vi "Main.vi"(11 "Module Admin":refnum<class "Delacor_lib_QMH_Cloneable Module Admin.lvclass">) -> ()   [LabVIEW 2020, in "Hardware Interface.lvlib"]
doc: "This template is based off of the Queued Message Handler design pattern and the Queued Message Handler project template that ships with LabVIEW.\n\nThe main difference is that the queue is private to this module and communication between modules is performed via Broadcast and Request events.\n\nRequest events are wrapped in public API methods and are handled in the Event Handling Loop (EHL) of this VI. Any module can register for Broadcast events sent by this module. The EHL generates messages based on user interface actions.\n\nThe Message Handling Loop (MHL) processes messages generated by the EHL, or by other messages. The messages are string values, so new messages can be added easily to the Message Cases case structure in the MHL. Each message cluster can also provide an optional value for Message Data, which is a variant that can be converted to whatever message-specific data is required.\n_____\nBased on Delacor QMH Project Template 5.0.0.82."
uses:
  Hardware Interface.lvlib
  <vilib>/Delacor/Delacor QMH/Libraries/Cloneable Module Admin_class/Delacor_lib_QMH_Cloneable Module Admin.lvclass
  C:/Program Files (x86)/National Instruments/LabVIEW 2020/vi.lib/Delacor/Delacor QMH/Libraries/Module Admin_class/Delacor_lib_QMH_Module Admin.lvclass
  Module Data--cluster.ctl
  MCU/MCU.lvclass
  <vilib>/Delacor/Delacor QMH/Libraries/Cloneable Module Admin_class/Delacor_lib_QMH_Cloneable Module Admin.lvclass/Delacor_lib_QMH_Cloneable Module Admin.ctl
  Stop Argument--cluster.ctl
  <vilib>/Delacor/Delacor QMH/Libraries/Message Queue_class/Delacor_lib_QMH_Message Queue.lvclass/Delacor_lib_QMH_Message Queue.ctl
  <vilib>/Delacor/Delacor QMH/Libraries/Module Admin_class/Delacor_lib_QMH_Module Admin.lvclass/Delacor_lib_QMH_Module Admin.ctl
  Serial Device Init Argument--cluster.ctl
  SetPort Argument--cluster.ctl
  <vilib>/Delacor/Delacor QMH/Libraries/Cloneable Module Admin_class/Delacor_lib_QMH_Get Module ID.vi
  <vilib>/Delacor/Delacor QMH/Libraries/Message Queue_class/Delacor_lib_QMH_Enqueue Message (Single).vi
  <vilib>/Delacor/Delacor QMH/Libraries/Module Admin_class/Delacor_lib_QMH_Get External Launch.vi
  <vilib>/Utility/error.llb/Error Cluster From Error Code.vi
  <vilib>/ErrorRing/Error Ring.xnode
  <vilib>/Delacor/Delacor QMH/Libraries/Message Queue_class/Delacor_lib_QMH_Message Queue.lvclass
panel:
  in  "Canal de ADC":u8
  in  "Update ADC":bool
  out "ADC":u16(knob) caption="Gauge" scale=0.0..4095.0
  in  "Pin a leer":u8
  in  "Adquirir Pin":bool
  out "Estado de pin":bool
  in  "Puerto a leer":u8
  in  "Adquirir Puerto":bool
  out "Salida de Puerto":bool[](array[boolean])
  in  "Entrada de Pin":bool
  in  "Escribir Pin":bool
  in  "Pin":u8
  in  "Puerto":u8
  in  "Escribir Puerto":bool
  in  "Entrada de Puerto":bool[](array[boolean])
  out "error out":errorcluster
  out "Status":string
  # "Hardware Abstraction Layer Example"
  # "Developed by Francisco Flores"
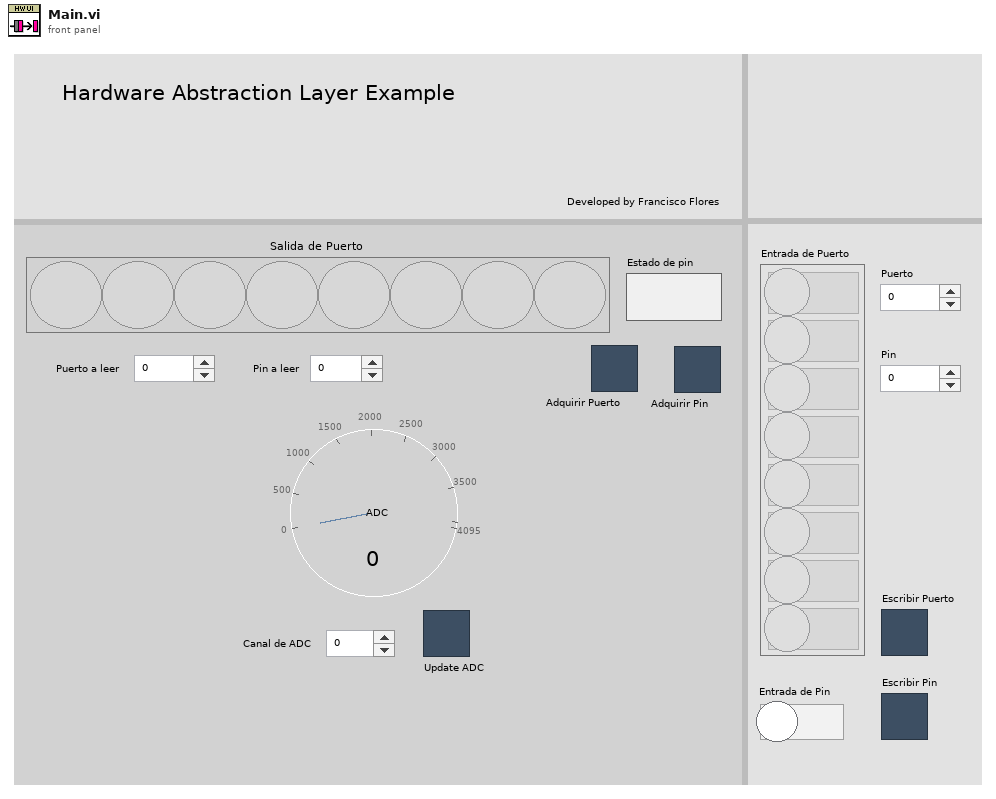
[diagram p1: front panel]
types:
  T1 = typedef "Hardware Interface.lvlib/Request Events--cluster.ctl" = cluster{"Stop Module":refnum<user-event>, "Show Panel":refnum<user-event>, "Hide Panel":refnum<user-event>, "Show Diagram":refnum<user-event>, "Get Module Execution Status":refnum<user-event>, "Serial Device Init":refnum<user-event>, "SetPort":refnum<user-event>}
  T2 = typedef "Hardware Interface.lvlib/Module Data--cluster.ctl" = cluster{"Status":string, "MCU.lvclass":refnum<class "MCU.lvclass">}
  T3 = enum32{"invalid lock state", "Not Locked", "Locked (No Password)", "Password-protected"}
  T4 = typedef "Hardware Interface.lvlib/Stop Argument--cluster.ctl" = cluster{"Module ID":i32, "Origin":string, "Exit via Stop Module Req?":bool, "Wait for Module to stop?":bool}
  T5 = typedef "Hardware Interface.lvlib/Serial Device Init Argument--cluster.ctl" = cluster{"Module ID":i32, "MCU.lvclass":refnum<class "MCU.lvclass">}
  T6 = typedef "Hardware Interface.lvlib/SetPort Argument--cluster.ctl" = cluster{"Module ID":i32, "Data":bool[], "Port":u8}
  T7 = enum32{"Invalid", "Standard", "Closed", "Hidden", "Minimized", "Maximized"}
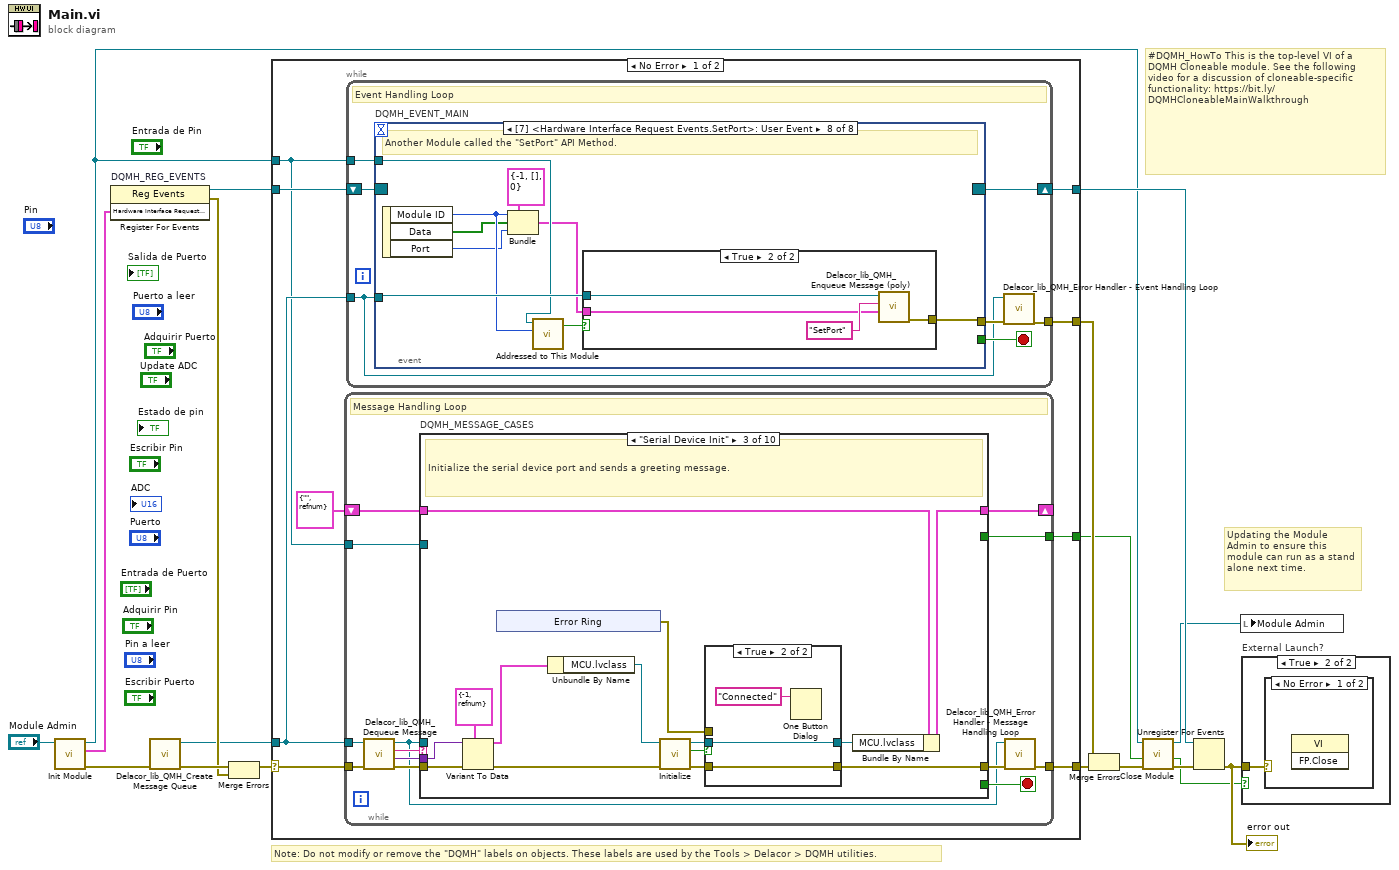
[diagram p0: block diagram]
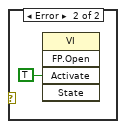
[diagram p3: hidden frame]
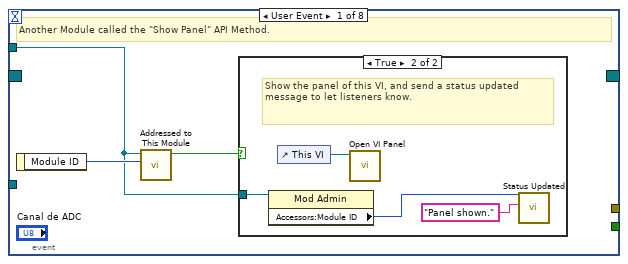
[diagram p4: hidden frame]
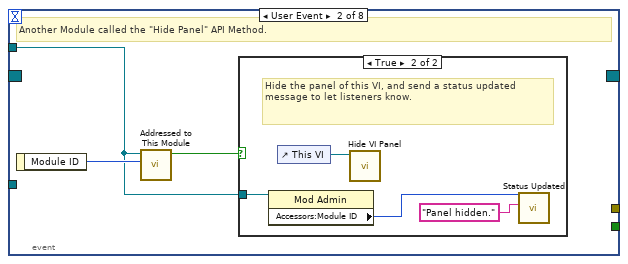
[diagram p6: hidden frame]
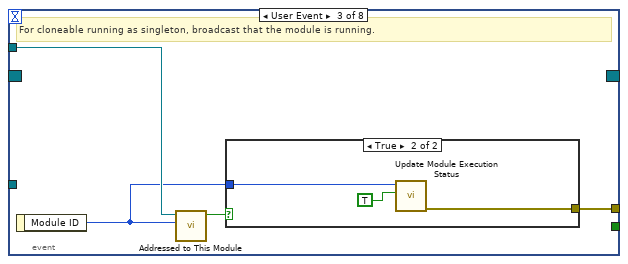
[diagram p8: hidden frame]
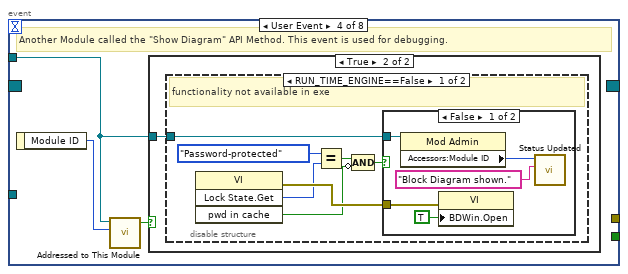
[diagram p10: hidden frame]
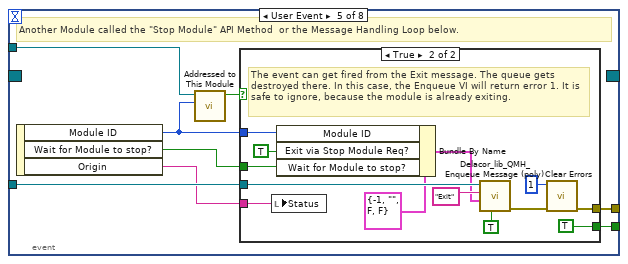
[diagram p14: hidden frame]
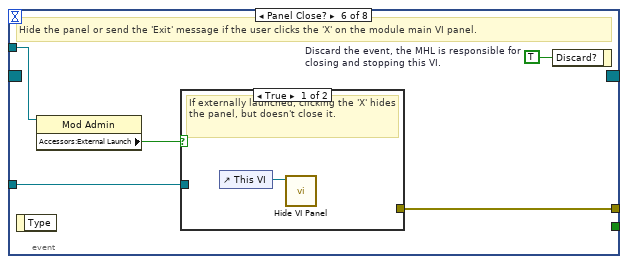
[diagram p16: hidden frame]
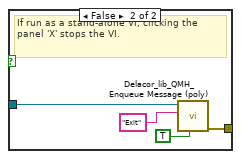
[diagram p17: hidden frame]
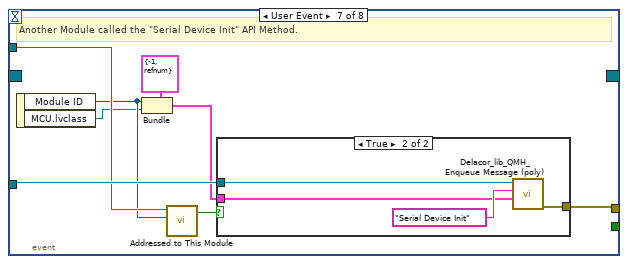
[diagram p18: hidden frame]
diagram:
  # "#DQMH_HowTo This is the top-level VI of a DQMH Cloneable module. See the following video for a discussion of cloneable-specific functionality: https://bit.ly/DQMHCloneableMainWalkthrough"
  # "Note: Do not modify or remove the \"DQMH\" labels on objects. These labels are used by the Tools > Delacor > DQMH utilities."
  # "Updating the Module Admin to ensure this module can run as a stand alone next time."
  n1 = call "Init Module.vi"("Cloneable Module Admin in"="Module Admin") -> ("error out"=w15:errorcluster, "Hardware Interface Request Events"=w7:T1, "Cloneable Module Admin out"=w4:refnum<class "Delacor_lib_QMH_Cloneable Module Admin.lvclass">)  [unwired: 8 in]
  n2 = register-events "DQMH_REG_EVENTS"(w7) -> (reference out=w8:refnum<event-registration>, error out=w10:errorcluster)  [unwired: 2 in]
  n3 = call <vilib>:"Delacor_lib_QMH_Create Message Queue.vi"("error in (no error)"=w15) -> ("error out"=w12:errorcluster, "Message Queue"=w6:refnum<class "Delacor_lib_QMH_Message Queue.lvclass">)  [unwired: 9 in]
  n4 = Merge Errors(w12, w10) -> (w11:errorcluster)
  n5 = case shown="No Error" w11 {
    selector: w11 -> [w25 w273]
    tunnel: [w27 w272] -> w16
    tunnel: [w24 w280] -> w9
    tunnel: w8 -> [w22 w280]
    tunnel: w6 -> [w21 w271]
    tunnel: [w26 _] -> w17
    tunnel: w4 -> [w20 w276]
    tunnel: [w19 _] -> w2
    frame No Error {
      n6 = while {
        tunnel: w21 -> [w131]
        shift-right: [w135] -> _
        shift-left: T2 {"Status"="", "MCU.lvclass"=refnum} ("Data Cluster") -> [w136]
        tunnel: w25 -> [w139]
        tunnel: [w137] -> w27
        tunnel: w20 -> [w129]
        tunnel: [w128] -> w19
        stop <- w134 stop-if-true
        # "Message Handling Loop"
        n7 = call-dynamic "Delacor_lib_QMH_Dequeue Message.vi"("error in (no error)"=w139, "Message Queue in"=w131) -> ("error out"=w138:errorcluster, "Message Data"=w132:variant, "Message"=w133:string, "Message Queue out"=w130:refnum<class "Delacor_lib_QMH_Message Queue.lvclass">)  [unwired: 6 in]
        n8 = case "DQMH_MESSAGE_CASES" shown="\"Serial Device Init\"" w133 {
          selector: w133 -> [_ _ _ _ _ _ _ _ _ w258]
          tunnel: w130 -> [_ _ _ _ _ _ w209 _ w248 _]
          tunnel: w138 -> [w158 w162 w176 w201 w204 w206 w218 w231 w254 w260]
          tunnel: [w156 w162 w166 w194 w203 w206 w214 w230 w251 w261] -> w140
          tunnel: w136 -> [w149 w161 w175 w197 w202 w205 w213 w228 w247 w259]
          tunnel: [w148 w161 w165 w196 w202 w205 w213 w228 w247 w259] -> w135
          tunnel: [_ _ _ _ _ _ _ _ w246 _] -> w134
          tunnel: w132 -> [_ _ w174 w200 _ _ w212 _ w244 _]
          tunnel: w129 -> [w143 _ _ _ _ _ w211 w226 w240 w256]
          tunnel: [_ _ _ _ _ _ _ _ w242 _] -> w128
          frame "Initialize" {
            w141 = "Initial Message" ("Initial Message")
            # "#CodeNeeded - Initialize the appearance of the front panel."
            # "#CodeNeeded - Initialize your state data here."
            # "Initialize - Any operation that needs to be done before the module can receive messages. Synchronize Caller Events.vi will inform Start Module.vi that the module has launched and is ready to receive messages. Module Did Init.vi will broadcast that the module initialized."
            n9 = call "Synchronize Caller Events.vi"("error in (no error)"=w158, "Module Admin"=w143) -> ("error out"=w157:errorcluster, "Module Admin out"=w142:refnum<class "Delacor_lib_QMH_Cloneable Module Admin.lvclass">)  [unwired: 8 in]
            n10 = property class="Mod Admin"(reference=w142) -> ("Accessors:Module ID"=w145:i32, "Accessors:External Launch"=w144:bool)  [unwired: 1 in, 2 out]
            n11 = call "Module Name--constant.vi"("Module ID"=w145) -> ("Module Name"=w153:string)  [unwired: 10 in]
            n12 = property class="VI"("Front Panel.Title"=w153) -> (reference out=w155:refnum<vi>, error out=w160:errorcluster)  [unwired: 2 in]
            n13 = Select(t=T7."Hidden" ("State"), s=w144, f=T7."Standard" ("State")) -> (s? t:f=w150:T7)
            n14 = invoke class="VI" method="FP.Open"(reference=w155, error in=w160, "State"=w150) -> (reference out=w154:refnum<vi>, error out=w159:errorcluster)  [unwired: 2 in, 3 out]
            n15 = call "Module Name--constant.vi"("Module ID"=w145) -> ("Module Name"=w146:string)  [unwired: 10 in]
            n16 = Bundle By Name(cluster=w149, "Status"=w141) -> (w148:T2)
            n17 = invoke class="VI" method="FP.Center"(reference=w154, error in=w159) -> ()  [unwired: 1 in, 3 out]
            n18 = call "Module Did Init.vi"("error in (no error)"=w157, "Initialized?"=TRUE, "Origin"=w146, "Module ID"=w145) -> ("error out"=w156:errorcluster)  [unwired: 7 in]
            "Status" <- w141
          }
          frame "--- Module Specific ---" {
            # "Separator -- The following cases handle messages specific to this Module."
          }
          frame "Serial Device Init" {
            # "Initialize the serial device port and sends a greeting message."
            n19 = Variant To Data(error in=w176, type=T5 {"Module ID"=-1, "MCU.lvclass"=refnum} ("Serial Device Init Argument"), Variant=w174) -> (data=w172:T5, error out=w171:errorcluster)
            n20 = xnode "Error Ring"() -> ("error out"=w163:errorcluster)
            n21 = Unbundle By Name(w172) -> ("MCU.lvclass"=w170:refnum<class "MCU.lvclass">)
            n22 = call-dynamic "Initialize.vi"("error in (no error)"=w171, "MCU in"=w170) -> ("error out"=w167:errorcluster, "Connected?"=w169:bool, "MCU out"=w168:refnum<class "MCU.lvclass">)  [unwired: 7 in]
            n23 = case shown="True" w169 {
              tunnel: w168 -> [_ w186]
              tunnel: w167 -> [_ w187]
              tunnel: [w184 w187] -> w166
              tunnel: [refnum<class "MCU.lvclass"> refnum ("MCU out") w186] -> w164
              tunnel: w163 -> [w184 _]
              frame False {
                n24 = One Button Dialog(message=" NotConnected") -> ()  [unwired: 1 in, 1 out]
              }
              frame True {
                n25 = One Button Dialog(message="Connected") -> ()  [unwired: 1 in, 1 out]
              }
            }
            n26 = Bundle By Name(cluster=w175, "MCU.lvclass"=w164) -> (w165:T2)
          }
          frame "SetPort" {
            # "Sets a specified value in a command to be sent to the HW."
            n27 = Variant To Data(error in=w201, type=T6 {"Module ID"=-1, "Data"=[], "Port"=0} ("SetPort Argument"), Variant=w200) -> (data=w198:T6, error out=w195:errorcluster)
            n28 = Unbundle By Name(w197) -> ("MCU.lvclass"=w193:refnum<class "MCU.lvclass">)
            n29 = Unbundle By Name(w198) -> ("Port"=w192:u8, "Data"=w191:bool[])
            n30 = Boolean Array To Number(Boolean array=w191) -> (number=w190:u32)
            n31 = To Unsigned Byte Integer(number=w190) -> (unsigned 8bit integer=w189:u8)
            n32 = call-dynamic "SetPort.vi"("error in (no error)"=w195, "Value"=w189, "Port"=w192, "MCU in"=w193) -> ("error out"=w194:errorcluster, "MCU out"=w188:refnum<class "MCU.lvclass">)  [unwired: 6 in]
            n33 = Bundle By Name(cluster=w197, "MCU.lvclass"=w188) -> (w196:T2)
          }
          frame "---Copy This Frame---" {
            # "Duplicate this frame when creating new messages.  Change this comment in the duplicated frame to describe this message."
            n34 = Merge Errors(w204) -> (w203:errorcluster)
          }
          frame "--- Exit and Error Handling---" {
            # "Separator - the following cases handle errors and exit messages."
          }
          frame "Error" {
            # "#CodeRecommended - If you ever change the name of this \"Error\" message, you'll need to update the name in the Check Loop Error.vi as well."
            # "#CodeRecommended - If the module is running in standalone mode (External Launch = FALSE), this code will pop up an error dialog and call the 'Exit' message if an error occurs. Add more fine-grained error handling here."
            # "Error - Check the error message data and respond accordingly. This message is sent by the \"Error Handler\" VIs at the end of each loop in this application."
            n35 = property class="Mod Admin"(reference=w211) -> ("Accessors:External Launch"=w210:bool, "Accessors:Module ID"=w207:i32)  [unwired: 1 in, 2 out]
            n36 = Variant To Data(error in=w218, type=errorcluster {"status"=FALSE, "code"=0, "source"=""} ("error constant"), Variant=w212) -> (data=w219:errorcluster, error out=w216:errorcluster)
            n37 = call "Module Name--constant.vi"("Module ID"=w207) -> ("Module Name"=w208:string)  [unwired: 10 in]
            n38 = call "Error Reported.vi"("Additional Information"=w208, "Error"=w219, "Module ID"=w207) -> ()  [unwired: 8 in, 1 out]
            n39 = case shown="False" w210 {
              tunnel: [w224 _] -> w215
              tunnel: w209 -> [w222 _]
              tunnel: w219 -> [w223 _]
              frame False {
                # "If the module is running standalone, then pop up an error dialog and call the \"Exit\" message."
                n40 = call <vilib>:"Simple Error Handler.vi"("error in (no error)"=w223) -> ()  [unwired: 4 in, 5 out]
                n41 = call-poly <vilib>:"Delacor_lib_QMH_Enqueue Message (poly).vi"("Priority Message? (F)"=TRUE, "Message"="Exit", "Message Queue in"=w222) -> ("error out"=w224:errorcluster)  [unwired: 7 in, 1 out]
              }
              frame True {
                # "If the module was launched externally, calling the Error Reported broadcast VI is the only action performed by the \"Error\" message. The module's caller can then process the error appropriately."
              }
            }
            n42 = Merge Errors(w216, w215) -> (w214:errorcluster)
            n43 = local write "error out"(w214) -> ()
          }
          frame "Simulate MHL Error" {
            # "#DQMH_HowTo The 'Simulate MHL Error' button  illustrates how the MHL handles errors. This event is instructional in nature and can be removed."
            # "Simulate an error occurring at the MHL"
            n44 = property class="Mod Admin"(reference=w226) -> ("Accessors:Module ID"=w227:i32)  [unwired: 1 in, 2 out]
            n45 = call "Module Name--constant.vi"("Module ID"=w227) -> ("Module Name"=w225:string)  [unwired: 10 in]
            n46 = xnode "Error Ring"("parameter 0"=w225) -> ("error out"=w229:errorcluster)
            n47 = Merge Errors(w231, w229) -> (w230:errorcluster)
          }
          frame "Exit" {
            w245 = 91  # 91: not all Exit messages will have an argument
            w246 = TRUE  # Stop the VI
            # "Release the message queue reference"
            # "#CodeNeeded - Add any required cleanup code here."
            # "Exit - Exit the application."
            n48 = Variant To Data(error in=w254, type=T4 {"Module ID"=-1, "Origin"="", "Exit via Stop Module Req?"=FALSE, "Wait for Module to stop?"=FALSE} ("Stop Argument"), Variant=w244) -> (data=w241:T4, error out=w249:errorcluster)
            n49 = call <vilib>:"Clear Errors.vi"("error in (no error)"=w249, "specific error code to clear (0: all)"=w245) -> ("error out"=w253:errorcluster)  [unwired: 4 in, 1 out]
            n50 = control-ref of="This VI"() -> (w239:refnum<vi>)
            n51 = call-dynamic "Delacor_lib_QMH_Release Message Queue.vi"("error in (no error)"=w253, "Message Queue"=w248) -> ("error out"=w252:errorcluster)  [unwired: 9 in]
            n52 = call "Handle Exit.vi"("Stop Argument"=w241, "Module Admin in"=w240, "VI reference"=w239) -> ("error out"=w250:errorcluster, "Wait for Stop?"=w242:bool)  [unwired: 7 in]
            n53 = Merge Errors(w252, w250) -> (w251:errorcluster)
          }
          frame Default {
            # "'Default' case only runs if there is a message that isn't defined in any of the other cases.  Output a programming error."
            n54 = property class="Mod Admin"(reference=w256) -> ("Accessors:Module ID"=w255:i32)  [unwired: 1 in, 2 out]
            n55 = call "Module Name--constant.vi"("Module ID"=w255) -> ("Module Name"=w257:string)  [unwired: 10 in]
            n56 = xnode "Error Ring"("parameter 0"=w258, "parameter 1"=w257) -> ("error out"=w262:errorcluster)
            n57 = Merge Errors(w260, w262) -> (w261:errorcluster)
          }
        }
        n58 = call-dynamic "Delacor_lib_QMH_Error Handler - Message Handling Loop.vi"("error in (no error)"=w140, "Message Queue in"=w130) -> ("dup error in"=w137:errorcluster)  [unwired: 8 in, 1 out]
      }
      n59 = while {
        tunnel: w21 -> [w28]
        shift-right: [w31] -> w24
        shift-left: w22 -> [w32]
        tunnel: [w33] -> w26
        tunnel: w20 -> [w29]
        stop <- w30 stop-if-true
        # "Event Handling Loop"
        n60 = event "DQMH_EVENT_MAIN" shown="[7] <Hardware Interface Request Events.SetPort>: User Event" {
          selector: w32 -> [_ _ _ _ _ _ _ _]
          dyn-events: [_ _ _ _ _ _ _ _] -> w31
          timeout: _ -> [_ _ _ _ _ _ _ _]
          tunnel: [_ _ _ _ w75 _ _ _] -> w30
          tunnel: w28 -> [_ _ _ _ w78 w94 w110 w123]
          tunnel: [_ _ w52 _ w79 w97 w103 w115] -> w34
          tunnel: w29 -> [w35 w42 w50 w56 w77 w95 w108 w121]
          event User Event {
            # "Another Module called the \"Show Panel\" API Method."
            n61 = event-data() -> ("Module ID"=w36:i32)  [unwired: 1 in]
            n62 = call "Addressed to This Module.vi"("Module ID from Argument"=w36, "Module Admin"=w35) -> ("Addressed to this instance?"=w37:bool)  [unwired: 8 in, 1 out]
            n63 = case shown="True" w37 {
              tunnel: w35 -> [_ w39]
              frame False {
              }
              frame True {
                # "Show the panel of this VI, and send a status updated message to let listeners know."
                n64 = property class="Mod Admin"(reference=w39) -> ("Accessors:Module ID"=w38:i32)  [unwired: 1 in, 2 out]
                n65 = control-ref of="This VI"() -> (w41:refnum<vi>)
                n66 = call "Open VI Panel.vi"("VI"=w41) -> ()  [unwired: 10 in, 1 out]
                n67 = call "Status Updated.vi"("Status"="Panel shown." ("format string"), "Module ID"=w38) -> ()  [unwired: 9 in, 1 out]
              }
            }
          }
          event User Event {
            # "Another Module called the \"Hide Panel\" API Method."
            n68 = event-data() -> ("Module ID"=w43:i32)  [unwired: 1 in]
            n69 = call "Addressed to This Module.vi"("Module ID from Argument"=w43, "Module Admin"=w42) -> ("Addressed to this instance?"=w44:bool)  [unwired: 8 in, 1 out]
            n70 = case shown="True" w44 {
              tunnel: w42 -> [_ w46]
              frame False {
              }
              frame True {
                # "Hide the panel of this VI, and send a status updated message to let listeners know."
                n71 = property class="Mod Admin"(reference=w46) -> ("Accessors:Module ID"=w45:i32)  [unwired: 1 in, 2 out]
                n72 = control-ref of="This VI"() -> (w48:refnum<vi>)
                n73 = call "Hide VI Panel.vi"("VI"=w48) -> ()  [unwired: 10 in, 1 out]
                n74 = call "Status Updated.vi"("Status"="Panel hidden." ("format string"), "Module ID"=w45) -> ()  [unwired: 9 in, 1 out]
              }
            }
          }
          event User Event {
            # "For cloneable running as singleton, broadcast that the module is running."
            n75 = event-data() -> ("Module ID"=w49:i32)  [unwired: 1 in]
            n76 = call "Addressed to This Module.vi"("Module ID from Argument"=w49, "Module Admin"=w50) -> ("Addressed to this instance?"=w51:bool)  [unwired: 8 in, 1 out]
            n77 = case shown="True" w51 {
              tunnel: [_ w55] -> w52
              tunnel: w49 -> [_ w54]
              frame False {
              }
              frame True {
                n78 = call "Update Module Execution Status.vi"("Running?"=TRUE, "Module ID"=w54) -> ("error out"=w55:errorcluster)  [unwired: 9 in]
              }
            }
          }
          event User Event {
            # "Another Module called the \"Show Diagram\" API Method. This event is used for debugging."
            n79 = event-data() -> ("Module ID"=w57:i32)  [unwired: 1 in]
            n80 = call "Addressed to This Module.vi"("Module ID from Argument"=w57, "Module Admin"=w56) -> ("Addressed to this instance?"=w58:bool)  [unwired: 8 in, 1 out]
            n81 = case shown="True" w58 {
              tunnel: w56 -> [_ w59]
              frame False {
              }
              frame True {
                n82 = disable-structure shown="RUN_TIME_ENGINE==False" {
                  disable-tunnel: w59 -> [w60 _]
                  frame condition #0 (active) {
                    # "functionality not available in exe"
                    n83 = invoke class="VI" method="Lock State.Get"() -> (error out=w66:errorcluster, "Get Lock State"=w65:T3, "pwd in cache"=w62:bool)  [unwired: 4 in, 1 out]
                    n84 = Equal?(x=T3."Password-protected", y=w65) -> (x = y?=w63:bool)
                    n85 = Compound Arithmetic op=AND(w63, invert w62) -> (w61:bool)
                    n86 = case shown="False" w61 {
                      tunnel: w66 -> [w71 _]
                      tunnel: w60 -> [w68 _]
                      frame False {
                        n87 = property class="Mod Admin"(reference=w68) -> ("Accessors:Module ID"=w67:i32)  [unwired: 1 in, 2 out]
                        n88 = property class="VI"(error in=w71, "BDWin.Open"=TRUE ("Block Diagram Window:Open")) -> ()  [unwired: 1 in, 2 out]
                        n89 = call "Status Updated.vi"("Status"="Block Diagram shown." ("format string"), "Module ID"=w67) -> ()  [unwired: 9 in, 1 out]
                      }
                      frame True {
                        # "Password-protected VI, and the password is not in the cache. Do not show the diagram."
                      }
                    }
                  }
                  frame condition #1 {
                  }
                }
              }
            }
          }
          event User Event {
            # "Another Module called the \"Stop Module\" API Method  or the Message Handling Loop below."
            n90 = event-data() -> ("Module ID"=w73:i32, "Wait for Module to stop?"=w74:bool, "Origin"=w72:string)  [unwired: 1 in]
            n91 = call "Addressed to This Module.vi"("Module ID from Argument"=w73, "Module Admin"=w77) -> ("Addressed to this instance?"=w76:bool)  [unwired: 8 in, 1 out]
            n92 = case shown="True" w76 {
              tunnel: [_ w91] -> w79
              tunnel: w78 -> [_ w87]
              tunnel: [_ TRUE] -> w75
              tunnel: w74 -> [_ w82]
              tunnel: w73 -> [_ w84]
              tunnel: w72 -> [_ w80]
              frame False {
              }
              frame True {
                # "The event can get fired from the Exit message. The queue gets destroyed there. In this case, the Enqueue VI will return error 1. It is safe to ignore, because the module is already exiting."
                n93 = local write "Status"(w80) -> ()
                n94 = Bundle By Name(cluster=T4 {"Module ID"=-1, "Origin"="", "Exit via Stop Module Req?"=FALSE, "Wait for Module to stop?"=FALSE} ("Stop Argument"), "Module ID"=w84, "Exit via Stop Module Req?"=TRUE, "Wait for Module to stop?"=w82) -> (w81:T4)
                n95 = call-poly <vilib>:"Delacor_lib_QMH_Enqueue Message (poly).vi"("Priority Message? (F)"=TRUE, "Message Data"=w81, "Message"="Exit", "Message Queue in"=w87) -> ("error out"=w92:errorcluster)  [unwired: 6 in, 1 out]
                n96 = call <vilib>:"Clear Errors.vi"("error in (no error)"=w92, "specific error code to clear (0: all)"=1) -> ("error out"=w91:errorcluster)  [unwired: 4 in, 1 out]
              }
            }
          }
          event Panel Close? {
            w96 = TRUE  # Discard the event, the MHL is responsible for closing and stopping this VI.
            # "Hide the panel or send the 'Exit' message if the user clicks the 'X' on the module main VI panel."
            n97 = event-data() -> ()  [unwired: 1 in, 1 out]
            n98 = property class="Mod Admin"(reference=w95) -> ("Accessors:External Launch"=w93:bool)  [unwired: 1 in, 2 out]
            n99 = case shown="True" w93 {
              tunnel: w94 -> [_ w101]
              tunnel: [_ w102] -> w97
              frame True {
                # "If externally launched, clicking the 'X' hides the panel, but doesn't close it."
                n100 = control-ref of="This VI"() -> (w98:refnum<vi>)
                n101 = call "Hide VI Panel.vi"("VI"=w98) -> ()  [unwired: 10 in, 1 out]
              }
              frame False {
                # "If run as a stand-alone VI, clicking the panel 'X' stops the VI."
                n102 = call-poly <vilib>:"Delacor_lib_QMH_Enqueue Message (poly).vi"("Priority Message? (F)"=TRUE, "Message"="Exit", "Message Queue in"=w101) -> ("error out"=w102:errorcluster)  [unwired: 7 in, 1 out]
              }
            }
            n103 = event-data("Discard?"=w96) -> ()  [unwired: 1 in, 1 out]
          }
          event User Event {
            # "Another Module called the \"Serial Device Init\" API Method."
            n104 = event-data() -> ("Module ID"=w105:i32, "MCU.lvclass"=w104:refnum<class "MCU.lvclass">)  [unwired: 1 in]
            n105 = Bundle(cluster=T5 {"Module ID"=-1, "MCU.lvclass"=refnum} ("Serial Device Init Argument"), "Module ID"=w105, "MCU.lvclass"=w104) -> (w106:T5)
            n106 = call "Addressed to This Module.vi"("Module ID from Argument"=w105, "Module Admin"=w108) -> ("Addressed to this instance?"=w109:bool)  [unwired: 8 in, 1 out]
            n107 = case shown="True" w109 {
              tunnel: w110 -> [_ w114]
              tunnel: w106 -> [_ w112]
              tunnel: [_ w111] -> w103
              frame False {
              }
              frame True {
                n108 = call-poly <vilib>:"Delacor_lib_QMH_Enqueue Message (poly).vi"("Message Data"=w112, "Message"="Serial Device Init", "Message Queue in"=w114) -> ("error out"=w111:errorcluster)  [unwired: 7 in, 1 out]
              }
            }
          }
          event User Event {
            # "Another Module called the \"SetPort\" API Method."
            n109 = event-data() -> ("Module ID"=w118:i32, "Data"=w117:bool[], "Port"=w116:u8)  [unwired: 1 in]
            n110 = Bundle(cluster=T6 {"Module ID"=-1, "Data"=[], "Port"=0} ("SetPort Argument"), "Module ID"=w118, "Data"=w117, "Port"=w116) -> (w119:T6)
            n111 = call "Addressed to This Module.vi"("Module ID from Argument"=w118, "Module Admin"=w121) -> ("Addressed to this instance?"=w122:bool)  [unwired: 8 in, 1 out]
            n112 = case shown="True" w122 {
              tunnel: w123 -> [_ w127]
              tunnel: w119 -> [_ w125]
              tunnel: [_ w124] -> w115
              frame False {
              }
              frame True {
                n113 = call-poly <vilib>:"Delacor_lib_QMH_Enqueue Message (poly).vi"("Message Data"=w125, "Message"="SetPort", "Message Queue in"=w127) -> ("error out"=w124:errorcluster)  [unwired: 7 in, 1 out]
              }
            }
          }
        }
        n114 = call-dynamic "Delacor_lib_QMH_Error Handler - Event Handling Loop.vi"("error in (no error)"=w34, "Message Queue in"=w28) -> ("dup error in"=w33:errorcluster)  [unwired: 8 in, 1 out]
      }
    }
    frame Error {
      n115 = call "Synchronize Caller Events.vi"("Module Admin"=w276) -> ("Module Admin out"=w275:refnum<class "Delacor_lib_QMH_Cloneable Module Admin.lvclass">)  [unwired: 9 in, 1 out]
      n116 = property class="Mod Admin"(reference=w275) -> ("Accessors:Module ID"=w274:i32)  [unwired: 1 in, 2 out]
      n117 = call-dynamic "Delacor_lib_QMH_Release Message Queue.vi"("error in (no error)"=w273, "Message Queue"=w271) -> ("error out"=w272:errorcluster)  [unwired: 9 in]
      n118 = call "Module Name--constant.vi"("Module ID"=w274) -> ("Module Name"=w279:string)  [unwired: 10 in]
      n119 = Format Into String(format string="An error occurred during initialization. %s is no longer running.", w279) -> (resulting string=w277:string)  [unwired: 2 in, 1 out]
      n120 = call "Error Reported.vi"("Additional Information"=w277, "Error"=w272, "Module ID"=w274) -> ()  [unwired: 8 in, 1 out]
    }
  }
  n121 = Merge Errors(w17, w16) -> (w18:errorcluster)
  n122 = call "Close Module.vi"("error in"=w18, "Wait for stop?"=w2, "Module Admin in"=w4) -> ("error out"=w14:errorcluster, "External Launch"=w1:bool, "Module Admin out"=w3:refnum<class "Delacor_lib_QMH_Cloneable Module Admin.lvclass">)  [unwired: 6 in]
  n123 = Unregister For Events(event registration refnum=w9, error in=w14) -> (error out=w13:errorcluster)
  "error out" <- w13
  n124 = local write "Module Admin"(w3) -> ()
  n125 = case "External Launch?" shown="True" w1 {
    tunnel: w13 -> [_ w281]
    frame False {
    }
    frame True {
      n126 = case shown="No Error" w281 {
        frame No Error {
          n127 = invoke class="VI" method="FP.Close"() -> ()  [unwired: 3 in, 3 out]
        }
        frame Error {
          n128 = invoke class="VI" method="FP.Open"("Activate"=TRUE ("Activate?")) -> ()  [unwired: 4 in, 5 out]
        }
      }
    }
  }
